vi "Do.vi"(8 "error in (no error)":errorcluster, 10 "Actor in":refnum<class "Actor.lvclass">, 11 "List of Measurements Message":refnum<class "List of Measurements Message.lvclass">) -> (0 "error out":errorcluster, 2 "Actor out":refnum<class "Actor.lvclass">)   [LabVIEW 2016, in "Controller UI.lvlib" / "List of Measurements Message.lvclass"]
uses:
  <userlib>/Common Components/Controller UI/Messages/List of Measurements Message/List of Measurements Message.lvclass
  <vilib>/ActorFramework/Actor/Actor.lvclass
  <userlib>/Common Components/Controller UI/Controller UI.lvclass
  C:/Program Files (x86)/National Instruments/LabVIEW 2016/vi.lib/ActorFramework/Actor/Actor.lvclass
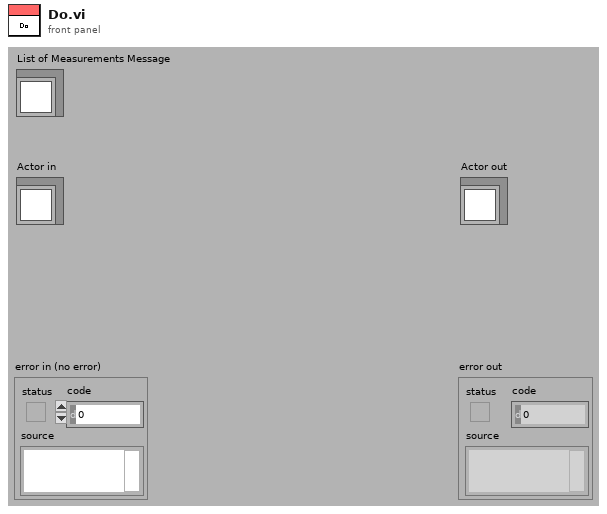
[diagram p1: front panel]
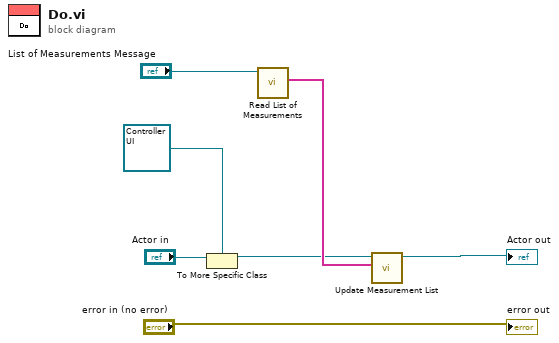
[diagram p0: block diagram]
diagram:
  n1 = To More Specific Class(target class=refnum<class "Controller UI.lvclass"> refnum ("UI.lvclass"), reference="Actor in") -> (specific class reference=w3:refnum<class "Controller UI.lvclass">)  [unwired: 1 in, 1 out]
  n2 = call <userlib>:"Read List of Measurements.vi"("List of Measurements Message in"="List of Measurements Message") -> ("List of Measurements"=w4:string[])  [unwired: 8 in, 2 out]
  n3 = call-dynamic "Update Measurement List.vi"("List of Measurements"=w4, "Operator UI in"=w3) -> ("Operator UI out"=→"Actor out":refnum<class "Controller UI.lvclass">)  [unwired: 8 in, 1 out]
  "error out" <- "error in (no error)"
